vi "DestroyPrivateEvents.vi"(8 "error in (no error)":errorcluster, 11 "MC":refnum<class "MC.lvclass">) -> (0 "error out":errorcluster, 3 "MC out":refnum<class "MC.lvclass">)   [LabVIEW 2017, in "MC.lvclass"]
doc: "JKI State Machine Objects (SMO) 1.0.2.13\nJKI - JKI\nCopyright (c) 2016, JKI"
uses:
  MC.lvclass
  <vilib>/JKI/JKI SMO/SMO/SMO.lvclass
panel:
  # "For instructions on how to use the JKI State Machine Objects, examples and video tutorials, visit:\nhttp://jki.net/state-machine-objects/\n\nJKI State Machine Objects™\nhttp://jki.net/state-machine-objects/\nCopyright (C) 2005-2015, JKI <info@jki.net>\nALL RIGHTS RESERVED"
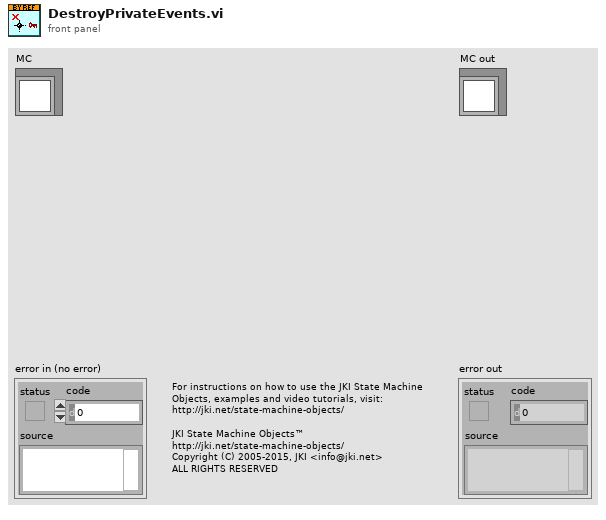
[diagram p1: front panel]
types:
  T1 = typedef "MC.lvclass/PrivateEvents--Cluster.ctl" = cluster{"New Value":refnum<user-event>}
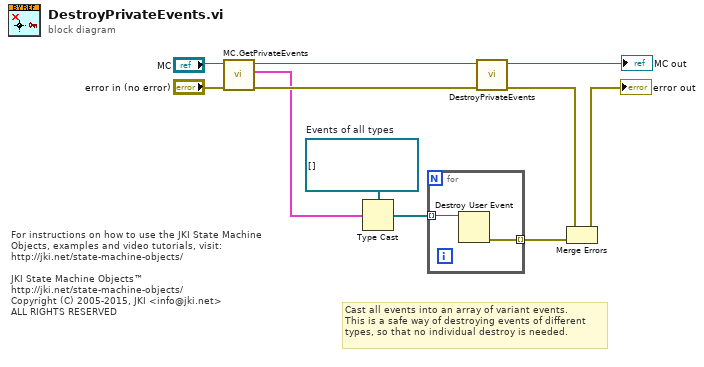
[diagram p0: block diagram]
diagram:
  w10 = refnum<user-event>[] []  # Events of all types
  # "For instructions on how to use the JKI State Machine Objects, examples and video tutorials, visit:\nhttp://jki.net/state-machine-objects/\n\nJKI State Machine Objects™\nhttp://jki.net/state-machine-objects/\nCopyright (C) 2005-2015, JKI <info@jki.net>\nALL RIGHTS RESERVED"
  # "Cast all events into an array of variant events.\nThis is a safe way of destroying events of different\ntypes, so that no individual destroy is needed."
  n1 = call "MC.GetPrivateEvents.vi"("error in (no error)"="error in (no error)", "MC"="MC") -> ("error out"=w4:errorcluster, "Private Events"=w3:T1, "MC out"=w5:refnum<class "MC.lvclass">)  [unwired: 7 in]
  n2 = Type Cast(type=w10, x=w3) -> (*(type *) &x=w9:refnum<user-event>[])
  n3 = for {
    tunnel: w9 -> [w13] mode=indexing
    tunnel: [w12] -> w8 mode=indexing
    n4 = Destroy User Event(user event=w13) -> (error out=w12:errorcluster)  [unwired: 1 in]
  }
  n5 = call-parent "DestroyPrivateEvents.vi"("error in (no error)"=w4, "SMO"=w5) -> ("error out"=w11:errorcluster, "SMO out"=→"MC out":refnum<class "MC.lvclass">)  [unwired: 8 in]
  n6 = Merge Errors(w11, w8) -> (→"error out":errorcluster)
